vi "Serialize - JSON.vi"(8 "error in":errorcluster, 11 "Data in":refnum<class "Data.lvclass">) -> (0 "error out":errorcluster, 2 "Serialized JSON":string, 3 "Data out":refnum<class "Data.lvclass">)   [LabVIEW 2014, in "Base Data Class.lvlib" / "Data.lvclass"]
uses:
  Data.lvclass
  Data.lvclass/Data.ctl
  Read Data ID.vi
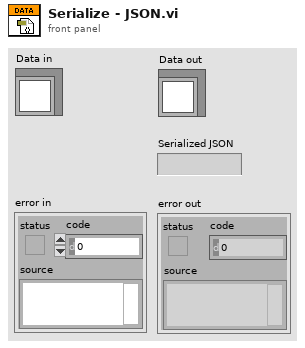
[diagram p1: front panel]
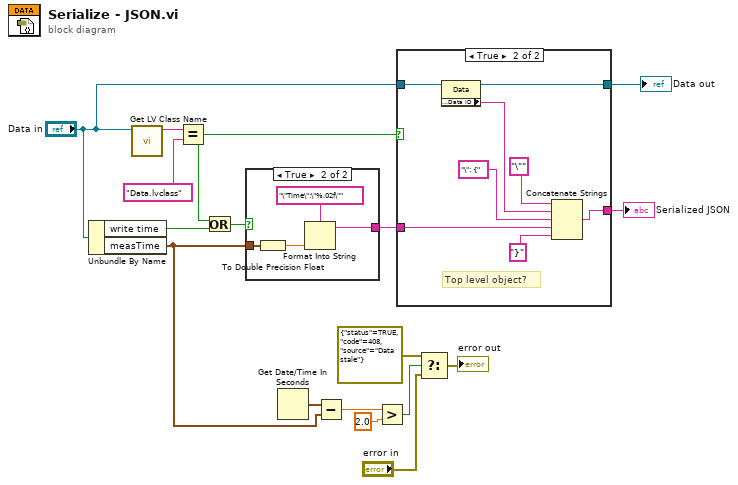
[diagram p0: block diagram]
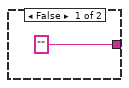
[diagram p3: hidden frame]
diagram:
  n1 = Unbundle By Name("Data in") -> ("write time"=w15:bool, "measTime"=w7:timestamp)
  n2 = call <vilib>:"Get LV Class Name.vi"("object"="Data in") -> ("class name"=w17:string)  [unwired: 9 in, 1 out]
  n3 = Equal?(x=w17, y="Data.lvclass") -> (x = y?=w13:bool)
  n4 = Or(x=w13, y=w15) -> (x .or. y?=w14:bool)
  n5 = case shown="True" w14 {
    tunnel: w7 -> [_ w22]
    tunnel: ["" w20] -> w11
    frame False {
    }
    frame True {
      n6 = To Double Precision Float(number=w22) -> (double precision float=w21:dbl)
      n7 = Format Into String(format string="\"Time\":\"%.02f\"", w21) -> (resulting string=w20:string)  [unwired: 2 in, 1 out]
    }
  }
  n8 = Get Date/Time In Seconds() -> (seconds since 1Jan1904=w8:timestamp)
  n9 = Subtract(x=w8, y=w7) -> (x-y=w6:dbl)
  n10 = Greater?(x=w6, y=2.0) -> (0:w4:bool)
  n11 = case shown="True" w13 {
    tunnel: "Data in" -> [w23 w32]
    tunnel: w11 -> [w24 w28]
    tunnel: [w24 w26] -> w10
    tunnel: [w23 w25] -> w9
    frame False {
    }
    frame True {
      # "Top level object?"
      n12 = property class="Data"(reference=w32) -> (reference out=w25:refnum<class "Data.lvclass">, "Accessors:Data ID"=w31:string)  [unwired: 1 in, 1 out]
      n13 = Concatenate Strings("\"" ("string"), w31, "\": {" ("string"), w28, "}" ("string")) -> (w26:string)
    }
  }
  "Data out" <- w9
  "Serialized JSON" <- w10
  n14 = Select(t=errorcluster {"status"=TRUE, "code"=408, "source"="Data stale"} ("error in"), s=w4, f="error in") -> (s? t:f=→"error out":errorcluster)
